vi "SendWaveFormServerSide.vi"() -> ()   [LabVIEW 2019]
uses:
  <vilib>/measure/NI_MABase.lvlib
panel:
  out "String":string
  out "error out":errorcluster
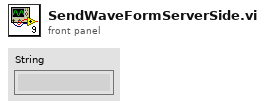
[diagram p1: front panel]
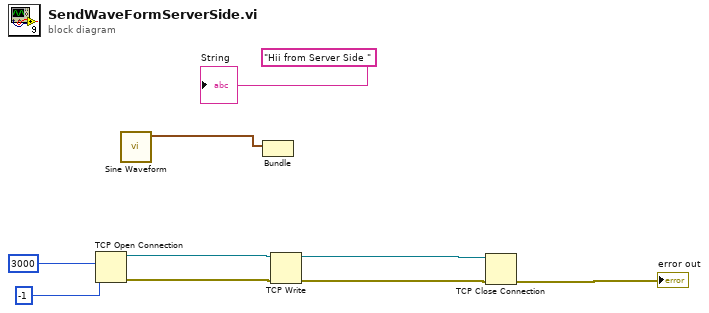
[diagram p0: block diagram]
diagram:
  n1 = TCP Open Connection(remote port or service name=u16 3000, timeout ms (60000)=-1) -> (connection ID=w7:refnum<k5>, error out=w5:errorcluster)  [unwired: 3 in]
  n2 = call <vilib>:"Sine Waveform.vi"() -> ("signal out"=w2:waveform(dbl))  [unwired: 10 in, 1 out]
  n3 = Bundle("signal out"=w2) -> ()  [unwired: 2 in, 1 out]
  n4 = TCP Write(connection ID=w7, error in (no error)=w5) -> (connection ID out=w6:refnum<k5>, error out=w4:errorcluster)  [unwired: 2 in, 1 out]
  n5 = TCP Close Connection(connection ID=w6, error in (no error)=w4) -> (error out=→"error out":errorcluster)  [unwired: 1 in, 1 out]
  "String" <- "Hii from Server Side " ("String")
